vi "Start Sync.vi"(8 "error in (no error)":errorcluster, 11 "gRPC Server in":refnum<class "GreeterService.lvclass">) -> (0 "error out":errorcluster, 3 "gRPC Server out":refnum<class "GreeterService.lvclass">)   [LabVIEW 2019, in "Generated_server.lvlib" / "GreeterService.lvclass"]
uses:
  GreeterService.lvclass
  GreeterService.lvclass/GreeterService.ctl
  RPC Messages/Greeter_res.ctl
  RPC Messages/Greeter_res_res_oneof/Greeter_res_res_oneof.lvclass
  RPC Messages/Greeter_req_req_oneof/Greeter_req_req_oneof.lvclass/Greeter_req_req_oneof.ctl
  RPC Messages/Greeter_res_res_oneof/Greeter_res_res_oneof.lvclass/Greeter_res_res_oneof.ctl
  RPC Messages/Greeter_req_req_oneof/Greeter_req_req_oneof.lvclass
  Generated_server.lvlib
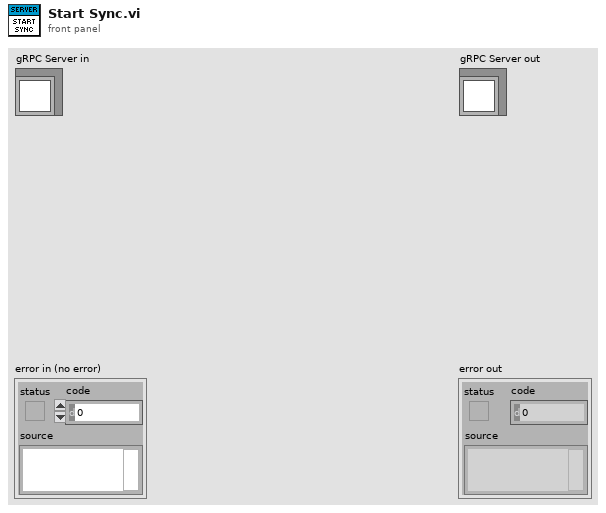
[diagram p1: front panel]
types:
  T1 = typedef "Generated_server.lvlib/Greeter_res.ctl" = cluster{"res_latitude":i32, "Greeter_res_res_oneof":refnum<class "Greeter_res_res_oneof.lvclass">}
  T2 = typedef "Generated_server.lvlib/GreeterService.lvclass/Server Internal UEs.ctl" = cluster{"GreeterService GetFeature Internal UE":refnum<user-event>}
  T3 = typedef "Generated_server.lvlib/GreeterService.lvclass/Server gRPC UEs.ctl" = cluster{"GreeterService GetFeature gRPC UE":refnum<user-event>}
  T4 = typedef "grpc-lvsupport-release.lvlib/grpcId.ctl" = u64
  T5 = typedef "Generated_server.lvlib/Greeter_req.ctl" = cluster{"req_latitude":i32, "Greeter_req_req_oneof":refnum<class "Greeter_req_req_oneof.lvclass">}
  T6 = typedef "grpc-lvsupport.lvlib/grpcId.ctl" = u64
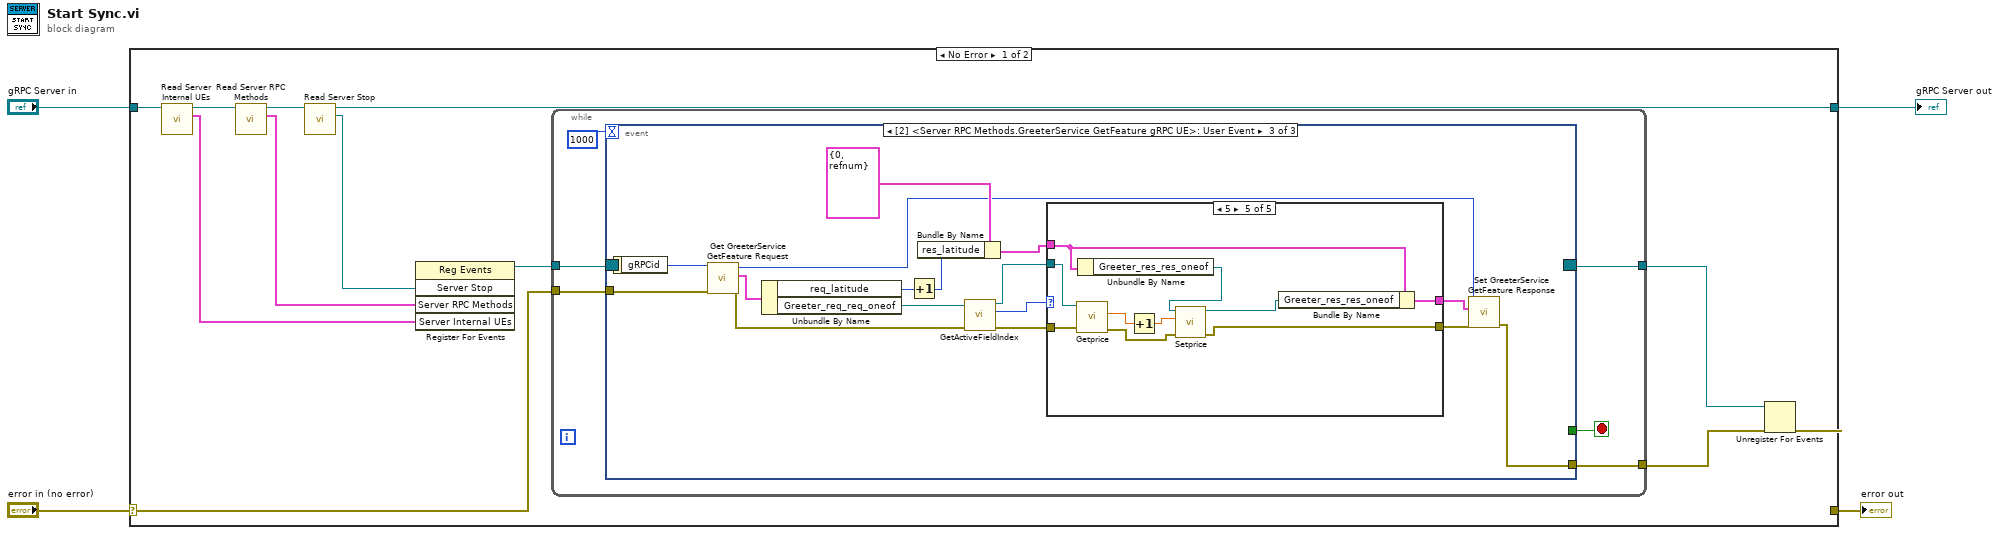
[diagram p0: block diagram]
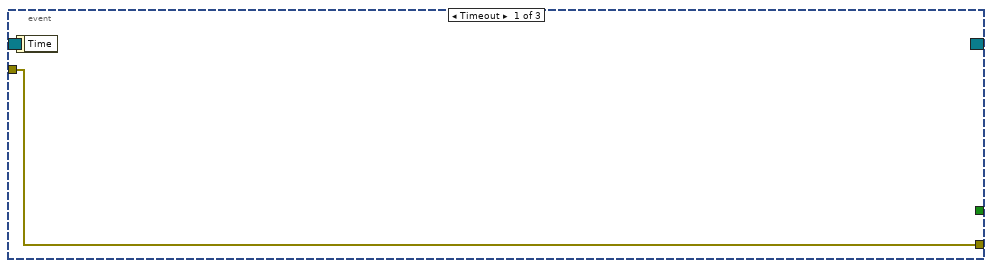
[diagram p2: hidden frame]
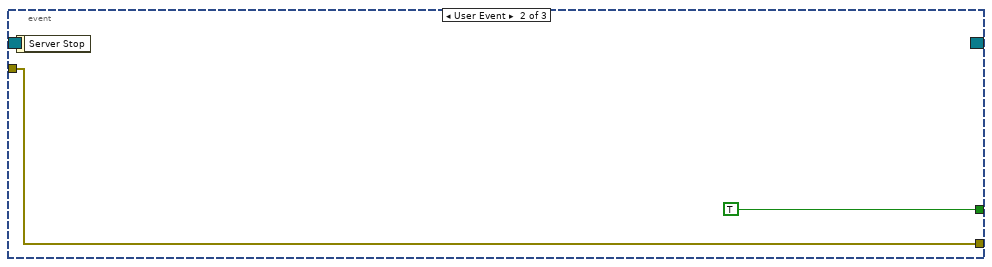
[diagram p3: hidden frame]
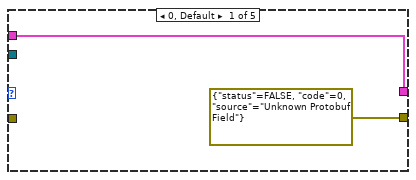
[diagram p4: hidden frame]
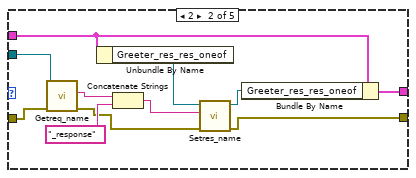
[diagram p5: hidden frame]
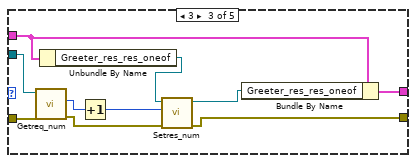
[diagram p6: hidden frame]
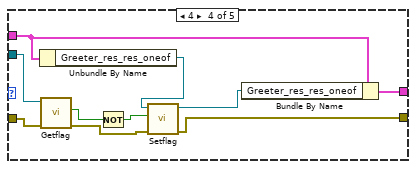
[diagram p7: hidden frame]
diagram:
  n1 = case shown="No Error" "error in (no error)" {
    selector: "error in (no error)" -> [w6 w86]
    tunnel: [w10 w86] -> w3
    tunnel: [w8 w85] -> w1
    tunnel: "gRPC Server in" -> [w16 w85]
    frame No Error {
      n2 = call "Read Server Internal UEs.vi"("SignalGeneratorService in"=w16) -> ("Server Internal UEs"=w14:T2, "SignalGeneratorService out"=w15:refnum<class "GreeterService.lvclass">)  [unwired: 8 in, 1 out]
      n3 = call "Read Server RPC Methods.vi"("SignalGeneratorService in"=w15) -> ("Server RPC Methods"=w9:T3, "SignalGeneratorService out"=w13:refnum<class "GreeterService.lvclass">)  [unwired: 8 in, 1 out]
      n4 = call-dynamic "Read Server Stop.vi"("iService in"=w13) -> ("Server Stop"=w7:refnum<user-event>, "iService out"=w8:refnum<class "GreeterService.lvclass">)  [unwired: 8 in, 1 out]
      n5 = register-events(w7, w9, w14) -> (reference out=w12:refnum<event-registration>)  [unwired: 2 in, 1 out]
      n6 = while {
        tunnel: w12 -> [w22]
        tunnel: [w20] -> w11
        tunnel: w6 -> [w18]
        tunnel: [w17] -> w5
        stop <- w21 stop-if-true
        n7 = event "RPC Methods Event Structure" shown="[2] <Server RPC Methods.GreeterService GetFeature gRPC UE>: User Event" {
          selector: w22 -> [_ _ _]
          dyn-events: [_ _ _] -> w20
          timeout: 1000 -> [_ _ _]
          tunnel: [_ TRUE _] -> w21
          tunnel: w18 -> [w23 w24 w27]
          tunnel: [w23 w24 w26] -> w17
          event Timeout {
            n8 = event-data() -> ()  [unwired: 1 in, 1 out]
          }
          event User Event {
            n9 = event-data() -> ()  [unwired: 1 in, 1 out]
          }
          event User Event {
            n10 = event-data() -> ("gRPCid"=w41:T4)  [unwired: 1 in]
            n11 = call "Get GreeterService GetFeature Request.vi"("error in (no error)"=w27, "gRPCid in"=w41) -> ("error out"=w38:errorcluster, "Message Data"=w40:T5, "gRPCid out"=w28:T6)  [unwired: 7 in]
            n12 = Unbundle By Name(w40) -> ("req_latitude"=w34:i32, "Greeter_req_req_oneof"=w39:refnum<class "Greeter_req_req_oneof.lvclass">)
            n13 = Increment(x=w34) -> (x+1=w33:i32)
            n14 = Bundle By Name(cluster=T1 {"res_latitude"=0, "Greeter_res_res_oneof"=refnum} ("Greeter_res"), "res_latitude"=w33) -> (w32:T1)
            n15 = call "GetActiveFieldIndex.vi"("error in (no error)"=w38, "OneOfTemplate in"=w39) -> ("error out"=w35:errorcluster, "Active Field Index"=w37:i32, "OneOfTemplate out"=w36:refnum<class "Greeter_req_req_oneof.lvclass">)  [unwired: 7 in]
            n16 = case shown="5" w37 {
              tunnel: w36 -> [_ w54 w62 w72 w83]
              tunnel: w35 -> [_ w53 w61 w71 w82]
              tunnel: w32 -> [w42 w47 w64 w74 w84]
              tunnel: [w42 w45 w63 w73 w76] -> w30
              tunnel: [errorcluster {"status"=FALSE, "code"=0, "source"="Unknown Protobuf Field"} ("error out") w44 w56 w65 w75] -> w31
              frame 0, Default {
              }
              frame 2 {
                n17 = call "Getreq_name.vi"("error in (no error)"=w53, "OneOfTemplate in"=w54) -> ("error out"=w48:errorcluster, "Get_Val"=w52:string)  [unwired: 7 in, 1 out]
                n18 = Unbundle By Name(w47) -> ("Greeter_res_res_oneof"=w50:refnum<class "Greeter_res_res_oneof.lvclass">)
                n19 = Concatenate Strings(w52, "_response" ("string")) -> (w49:string)
                n20 = call "Setres_name.vi"("error in (no error)"=w48, "Set_Val"=w49, "OneOfTemplate in"=w50) -> ("error out"=w44:errorcluster, "OneOfTemplate out"=w46:refnum<class "Greeter_res_res_oneof.lvclass">)  [unwired: 7 in]
                n21 = Bundle By Name(cluster=w47, "Greeter_res_res_oneof"=w46) -> (w45:T1)
              }
              frame 3 {
                n22 = call "Getreq_num.vi"("error in (no error)"=w61, "OneOfTemplate in"=w62) -> ("error out"=w55:errorcluster, "Get_Val"=w60:i32)  [unwired: 7 in, 1 out]
                n23 = Unbundle By Name(w64) -> ("Greeter_res_res_oneof"=w58:refnum<class "Greeter_res_res_oneof.lvclass">)
                n24 = Increment(x=w60) -> (x+1=w59:i32)
                n25 = call "Setres_num.vi"("error in (no error)"=w55, "Set_Val"=w59, "OneOfTemplate in"=w58) -> ("error out"=w56:errorcluster, "OneOfTemplate out"=w57:refnum<class "Greeter_res_res_oneof.lvclass">)  [unwired: 7 in]
                n26 = Bundle By Name(cluster=w64, "Greeter_res_res_oneof"=w57) -> (w63:T1)
              }
              frame 4 {
                n27 = Unbundle By Name(w74) -> ("Greeter_res_res_oneof"=w68:refnum<class "Greeter_res_res_oneof.lvclass">)
                n28 = call "Getflag.vi"("error in (no error)"=w71, "OneOfTemplate in"=w72) -> ("error out"=w67:errorcluster, "Get_Val"=w70:bool)  [unwired: 7 in, 1 out]
                n29 = Not(x=w70) -> (.not. x?=w69:bool)
                n30 = call "Setflag.vi"("error in (no error)"=w67, "Set_Val"=w69, "OneOfTemplate in"=w68) -> ("error out"=w65:errorcluster, "OneOfTemplate out"=w66:refnum<class "Greeter_res_res_oneof.lvclass">)  [unwired: 7 in]
                n31 = Bundle By Name(cluster=w74, "Greeter_res_res_oneof"=w66) -> (w73:T1)
              }
              frame 5 {
                n32 = call "Getprice.vi"("error in (no error)"=w82, "OneOfTemplate in"=w83) -> ("error out"=w78:errorcluster, "Get_Val"=w80:sgl)  [unwired: 7 in, 1 out]
                n33 = Unbundle By Name(w84) -> ("Greeter_res_res_oneof"=w79:refnum<class "Greeter_res_res_oneof.lvclass">)
                n34 = Increment(x=w80) -> (x+1=w81:sgl)
                n35 = call "Setprice.vi"("error in (no error)"=w78, "Set_Val"=w81, "OneOfTemplate in"=w79) -> ("error out"=w75:errorcluster, "OneOfTemplate out"=w77:refnum<class "Greeter_res_res_oneof.lvclass">)  [unwired: 7 in]
                n36 = Bundle By Name(cluster=w84, "Greeter_res_res_oneof"=w77) -> (w76:T1)
              }
            }
            n37 = call "Set GreeterService GetFeature Response.vi"("error in (no error)"=w31, "Message Data"=w30, "gRPCid in"=w28) -> ("error out"=w26:errorcluster)  [unwired: 8 in]
          }
        }
      }
      n38 = Unregister For Events(event registration refnum=w11, error in=w5) -> (error out=w10:errorcluster)
    }
    frame Error {
    }
  }
  "error out" <- w3
  "gRPC Server out" <- w1
